vi "Elevator_Set.vi"() -> ()   [LabVIEW 2019]
uses:
  Climb_Elevator_Control_States.ctl
  Globals/Climb_Globals.vi
  Globals/Sensor_Values.vi
panel:
  in  "Up_Threshold":dbl
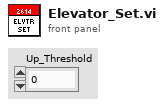
[diagram p1: front panel]
types:
  T1 = typedef "Climb_Elevator_Control_States.ctl" = enum16{"No-Op", "Brake", "Going_Up", "Going_Down", "Manual_PercentVoltage", "Manual_SpeedControl"}
  T2 = typedef "Climb_Elevator_Cluster.ctl" = cluster{"Extend?":bool, "Elevator_Throttle":dbl, "Control_States":T1}
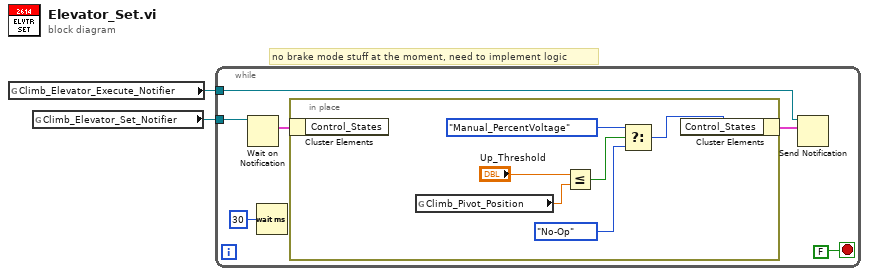
[diagram p0: block diagram]
diagram:
  # "no brake mode stuff at the moment, need to implement logic"
  n1 = global read "Climb_Globals.vi" "Climb_Elevator_Execute_Notifier"() -> (w1:refnum<notifier>)
  n2 = global read "Climb_Globals.vi" "Climb_Elevator_Set_Notifier"() -> (w2:refnum<notifier>)
  n3 = while {
    tunnel: w2 -> [w7]
    tunnel: w1 -> [w6]
    stop <- FALSE stop-if-true
    n4 = Wait on Notification(notifier=w7) -> (notification=w5:T2)  [unwired: 3 in, 3 out]
    n5 = Wait (ms)(milliseconds to wait=u32 30) -> ()  [unwired: 1 out]
    n6 = in-place {
      n7 = in-place-cluster #1(w5) -> ()  [unwired: 1 out]
      n8 = global read "Sensor_Values.vi" "Climb_Pivot_Position"() -> (w12:dbl)
      n9 = Less Or Equal?(x="Up_Threshold", y=w12) -> (x <= y?=w11:bool)
      n10 = Select(t=Climb_Elevator_Control_States."Manual_PercentVoltage" ("Control_States"), s=w11, f=Climb_Elevator_Control_States."No-Op" ("Control_States")) -> (s? t:f=w9:T1)
      n11 = in-place-cluster #1("Control_States"=w9) -> (w4:T2)
    }
    n12 = Send Notification(notification=w4, notifier=w6) -> ()  [unwired: 1 in, 2 out]
  }
